vi "Encoders.vi"(0 "Reset Encoders?":bool) -> (3 "Total Distance":dbl, 4 "Avg Rate":dbl, 5 "X Distance":dbl, 6 "Y Distance":dbl)   [LabVIEW 2017, in "Support Code.lvlib"]
uses:
  Support Code.lvlib
panel:
  in  "Manual Reset":bool
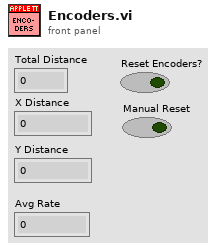
[diagram p1: front panel]
types:
  T1 = typedef "WPI_EncoderDevRef.ctl" = cluster{"DevStatus":errorcluster, "EncoderIndex":T2, "CounterIndex":T3, "DistancePerCount":dbl, "Decoding Type":T4}
  T2 = typedef "FPGA_EncoderIdx.ctl" = enum8{"Enc 0", "Enc 1", "Enc 2", "Enc 3", "Enc 4", "Enc 5", "Enc 6", "Enc 7", "Invalid"}
  T3 = typedef "FPGA_CounterCtrSystemIndex.ctl" = enum8{"Ctr 0", "Ctr 1", "Ctr 2", "Ctr 3", "Ctr 4", "Ctr 5", "Ctr 6", "Ctr 7", "Invalid"}
  T4 = typedef "WPI_EncoderType.ctl" = enum16{"1x", "2x", "4x"}
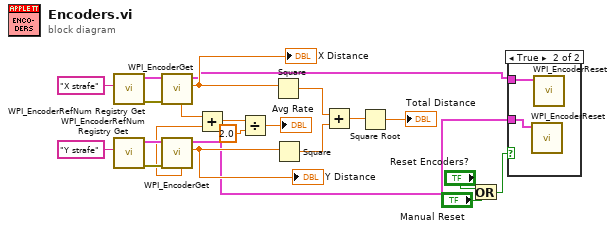
[diagram p0: block diagram]
diagram:
  n1 = call <vilib>:"WPI_EncoderRefNum Registry Get.vi"("refnum name"="X strafe") -> ("error out"=w22:errorcluster, "EncoderDevRef"=w21:T1)  [unwired: 9 in]
  n2 = call <vilib>:"WPI_EncoderRefNum Registry Get.vi"("refnum name"="Y strafe") -> ("error out"=w17:errorcluster, "EncoderDevRef"=w18:T1)  [unwired: 9 in]
  n3 = call <vilib>:"WPI_EncoderGet.vi"("error in (no error)"=w22, "EncoderDevRef"=w21) -> ("Distance"=w12:dbl, "EncoderDevRef"=w4:T1, "Rate"=w9:dbl)  [unwired: 4 in, 3 out]
  "X Distance" <- w12
  n4 = call <vilib>:"WPI_EncoderGet.vi"("error in (no error)"=w17, "EncoderDevRef"=w18) -> ("Distance"=w16:dbl, "EncoderDevRef"=w5:T1, "Rate"=w8:dbl)  [unwired: 4 in, 3 out]
  "Y Distance" <- w16
  n5 = Add(x=w9, y=w8) -> (x+y=w10:dbl)
  n6 = Divide(x=w10, y=2.0) -> (x/y=→"Avg Rate":dbl)
  n7 = Square(x=w12) -> (x^2=w14:dbl)
  n8 = Square(x=w16) -> (x^2=w13:dbl)
  n9 = Add(x=w14, y=w13) -> (x+y=w15:dbl)
  n10 = Square Root(x=w15) -> (sqrt(x)=→"Total Distance":dbl)
  n11 = Or(x="Reset Encoders?", y="Manual Reset") -> (x .or. y?=w3:bool)
  n12 = case shown="True" w3 {
    tunnel: w5 -> [_ w23]
    tunnel: w4 -> [_ w24]
    frame False {
    }
    frame True {
      n13 = call <vilib>:"WPI_EncoderReset.vi"("EncoderDevRef"=w23) -> ()  [unwired: 9 in, 2 out]
      n14 = call <vilib>:"WPI_EncoderReset.vi"("EncoderDevRef"=w24) -> ()  [unwired: 9 in, 2 out]
    }
  }
